vi "execute.vi"(8 "error in (no error)":errorcluster, 11 "command in":refnum<class "command_generic.lvclass">) -> (0 "error out":errorcluster, 3 "command out":refnum<class "command_generic.lvclass">)   [LabVIEW 2015, in "command_generic.lvclass"]
uses:
  command_generic.lvclass
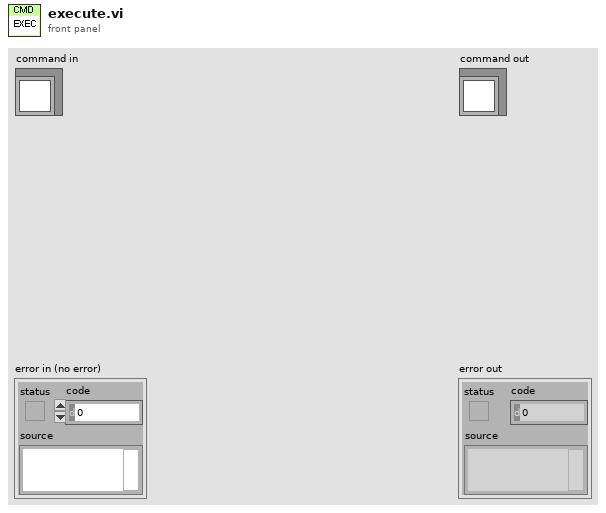
[diagram p1: front panel]
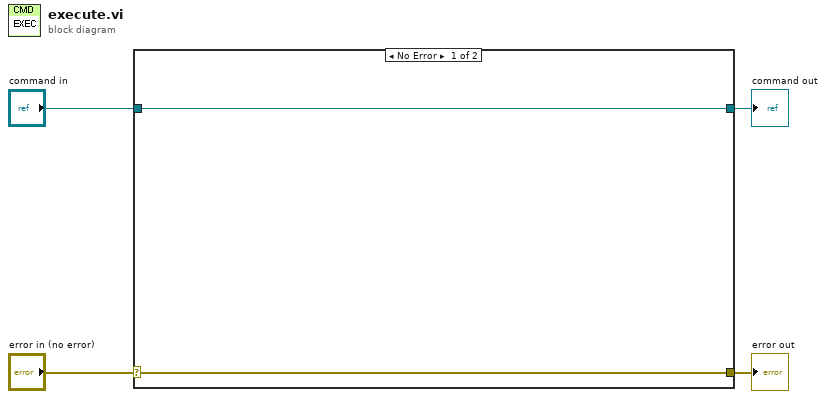
[diagram p0: block diagram]
diagram:
  n1 = case shown="No Error" "error in (no error)" {
    selector: "error in (no error)" -> [w5 w8]
    tunnel: [w5 w8] -> w3
    tunnel: [w6 w7] -> w1
    tunnel: "command in" -> [w6 w7]
    frame No Error {
    }
    frame Error {
    }
  }
  "error out" <- w3
  "command out" <- w1
